vi "attach_observer.vi"(8 "error in (no error)":errorcluster, 10 "top-level component type":T1, 11 "GenericToplevelComponent in":refnum<class "GenericToplevelComponent.lvclass">) -> (0 "error out":errorcluster, 3 "GenericToplevelComponent out":refnum<class "GenericToplevelComponent.lvclass">)   [LabVIEW 2010, in "GenericToplevelComponent.lvclass"]
uses:
  GenericToplevelComponent.lvclass
  enumerations/top-level_component_type_enum.ctl
  GenericToplevelComponent.lvclass/GenericToplevelComponent.ctl
  ErrorController/ErrorController/class_data.vi
  ErrorController/ErrorController/ErrorController.lvclass
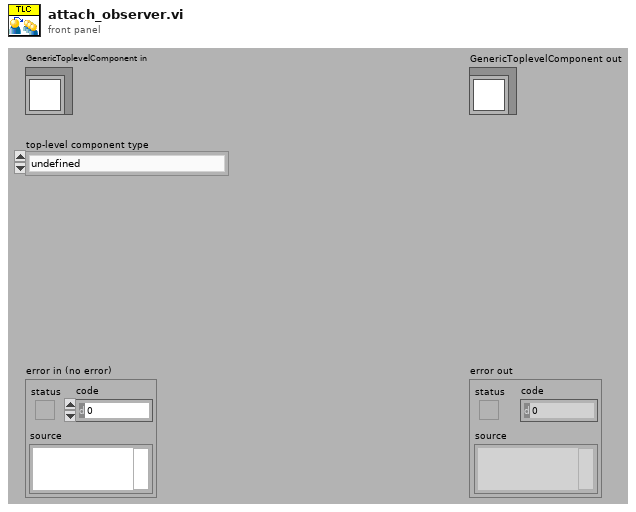
[diagram p1: front panel]
types:
  T1 = typedef "top-level_component_type_enum.ctl" = enum16{"undefined", "ImagingMode", "ScanHead", "DAQ", "ImageAssembler", "Display", "DataCollection", "Analyser", "Stimulator", "ExperimentController", "Instrument", "Stage"}
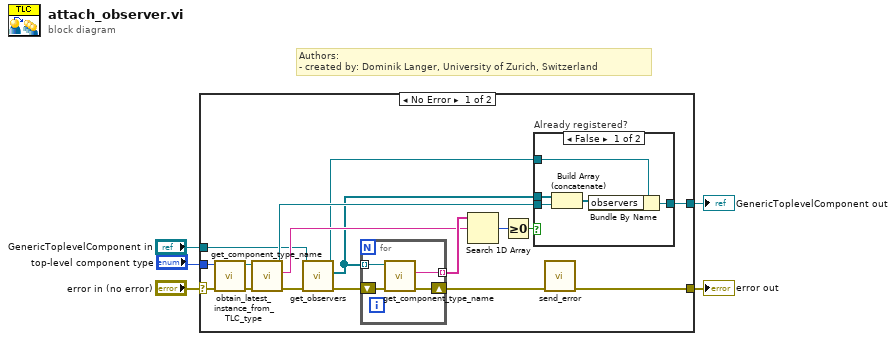
[diagram p0: block diagram]
diagram:
  # "Authors: \n- created by: Dominik Langer, University of Zurich, Switzerland"
  n1 = case shown="No Error" "error in (no error)" {
    selector: "error in (no error)" -> [w13 w34]
    tunnel: [w16 w34] -> w4
    tunnel: [w15 w33] -> w2
    tunnel: "GenericToplevelComponent in" -> [w7 w33]
    tunnel: "top-level component type" -> [w14 _]
    frame No Error {
      n2 = call "obtain_latest_instance_from_TLC_type.vi"("error in (no error)"=w13, "top-level component type"=w14) -> ("error out"=w12:errorcluster, "GenericToplevelComponent.lvclass"=w11:refnum<class "GenericToplevelComponent.lvclass">)  [unwired: 8 in]
      n3 = call-dynamic "get_component_type_name.vi"("error in (no error)"=w12, "GenericPlugin in"=w11) -> ("error out"=w9:errorcluster, "component type"=w21:string, "GenericPlugin out"=w18:refnum<class "GenericToplevelComponent.lvclass">)  [unwired: 7 in]
      n4 = call-dynamic "get_observers.vi"("error in (no error)"=w9, "GenericToplevelComponent in"=w7) -> ("error out"=w8:errorcluster, "observers"=w10:refnum<class "GenericToplevelComponent.lvclass">[], "GenericToplevelComponent out"=w6:refnum<class "GenericToplevelComponent.lvclass">)  [unwired: 7 in]
      n5 = for {
        shift-right: [w31] -> w17
        shift-left: w8 -> [w32]
        tunnel: w10 -> [w30] mode=indexing
        tunnel: [w29] -> w22 mode=indexing
        n6 = call-dynamic "get_component_type_name.vi"("error in (no error)"=w32, "GenericPlugin in"=w30) -> ("error out"=w31:errorcluster, "component type"=w29:string)  [unwired: 7 in, 1 out]
      }
      n7 = Search 1D Array(1D array=w22, element=w21) -> (index of element=w20:i32)  [unwired: 1 in]
      n8 = Greater Or Equal To 0?(x=w20) -> (x >= 0?=w19:bool)
      n9 = case "Already registered?" shown="False" w19 {
        tunnel: w10 -> [w27 _]
        tunnel: w18 -> [w26 _]
        tunnel: w6 -> [w24 w28]
        tunnel: [w23 w28] -> w15
        frame False {
          n10 = Build Array (concatenate)(w27, w26) -> (w25:refnum<class "GenericToplevelComponent.lvclass">[])
          n11 = Bundle By Name(cluster=w24, "observers"=w25) -> (w23:refnum<class "GenericToplevelComponent.lvclass">)
        }
        frame True {
        }
      }
      n12 = call "send_error.vi"("error in (no error)"=w17) -> ("error out"=w16:errorcluster)  [unwired: 10 in]
    }
    frame Error {
    }
  }
  "error out" <- w4
  "GenericToplevelComponent out" <- w2
